vi "FTW-Actor-Broker-Initialize.vi"(0 "FTW Message Broker":refnum<class "FTW-Actor-Broker.lvclass">, 5 "Initialized Response":refnum<class "FTW-Container.lvclass">, 11 "error in":errorcluster) -> (4 "FTW Message Broker out":refnum<class "FTW-Actor-Broker.lvclass">, 6 "Observer":refnum<event-registration>, 15 "error out":errorcluster)   [LabVIEW 2014, in "FTW-Actor-Broker.lvclass"]
uses:
  FTW-Actor-Broker.lvclass
  Container/FTW-Container.lvclass
  Messaging/Message/FTW-Message.lvclass
panel:
  # "Inputs"
  # "Outputs"
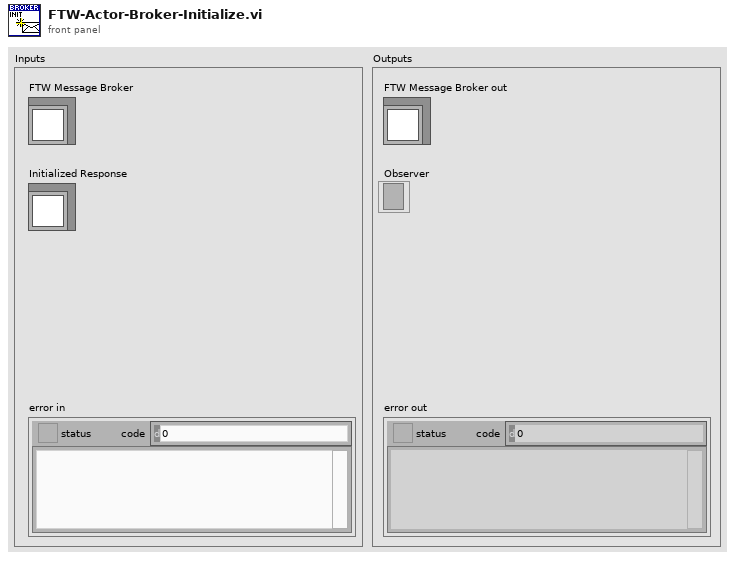
[diagram p1: front panel]
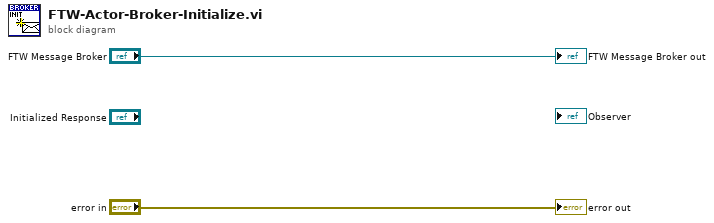
[diagram p0: block diagram]
diagram:
  "error out" <- "error in"
  "FTW Message Broker out" <- "FTW Message Broker"
